vi "U8 to U16 data.vi"(8 "Error In":errorcluster, 10 "Characteristic value":u8[](array[numeric])) -> (0 "Error Out":errorcluster, 2 "Characteristic value":u16[](array[numeric]))   [LabVIEW 2016]
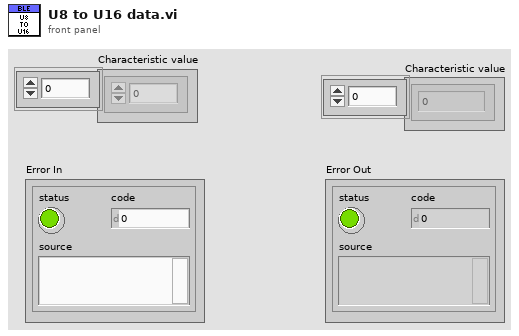
[diagram p1: front panel]
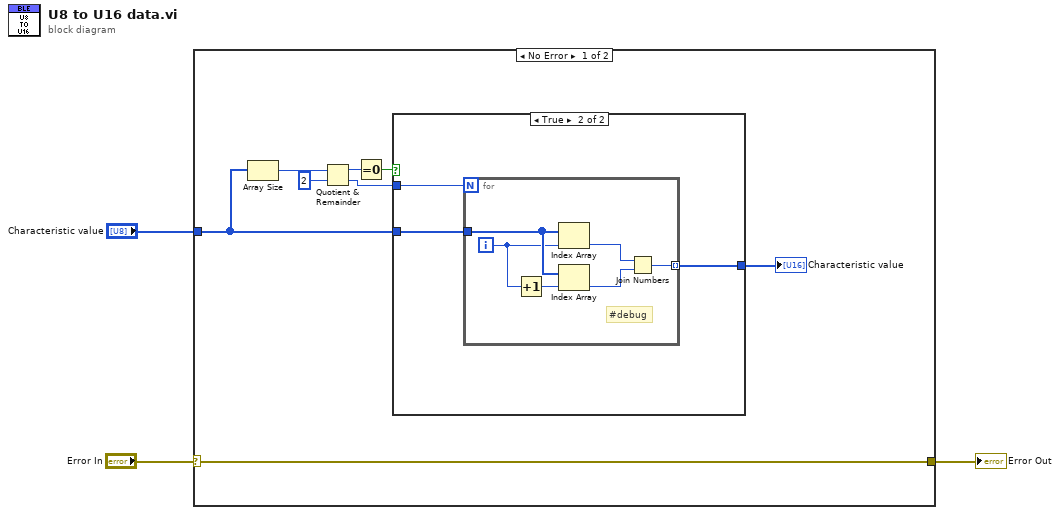
[diagram p0: block diagram]
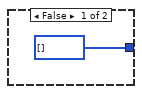
[diagram p2: hidden frame]
diagram:
  n1 = case shown="No Error" "Error In" {
    selector: "Error In" -> [w4 w22]
    tunnel: "Characteristic value" -> [w11 _]
    tunnel: [w4 w22] -> w1
    frame No Error {
      n2 = Array Size(array=w11) -> (size(s)=w10:i32)
      n3 = Quotient & Remainder(x=w10, y=2) -> (x-y*floor(x/y)=w7:i32, floor(x/y)=w6:i32)
      n4 = Equal To 0?(x=w7) -> (x = 0?=w8:bool)
      n5 = case shown="True" w8 {
        tunnel: w11 -> [_ w15]
        tunnel: w6 -> [_ w14]
        tunnel: [u16[] [] w13] -> w5
        frame False {
        }
        frame True {
          n6 = for {
            N: w14 -> [_]
            tunnel: w15 -> [w21]
            tunnel: [w16] -> w13 mode=indexing
            i -> [w19]
            # "#debug"
            n7 = Increment(x=w19) -> (x+1=w20:i32)
            n8 = Index Array(array=w21, index=w19) -> (element=w18:u8)
            n9 = Index Array(array=w21, index=w20) -> (element=w17:u8)
            n10 = Join Numbers(hi=w18, lo=w17) -> ((hi.lo)=w16:u16)
          }
        }
      }
      "Characteristic value" <- w5
    }
    frame Error {
    }
  }
  "Error Out" <- w1
